vi "Web Server Startup.vi"(6 "LabVIEW Web Service":refnum<class "Web Service.lvclass">) -> ()   [LabVIEW 2026]
uses:
  <vilib>/wsapi/Web Service.lvclass
panel:
  # "Use the web service input terminal to call the VIs on the Service subpalette of the Web Services palette. Do not remove it from the connector pane unless you don't need access to the palette."
  # "Any additional terminals added to the connector pane of a startup VI will be ignored."
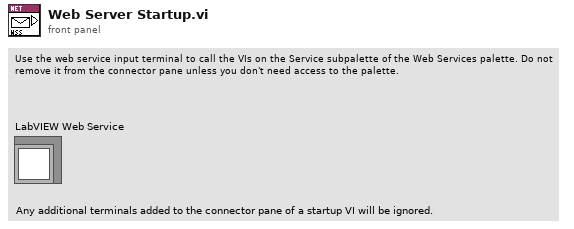
[diagram p1: front panel]
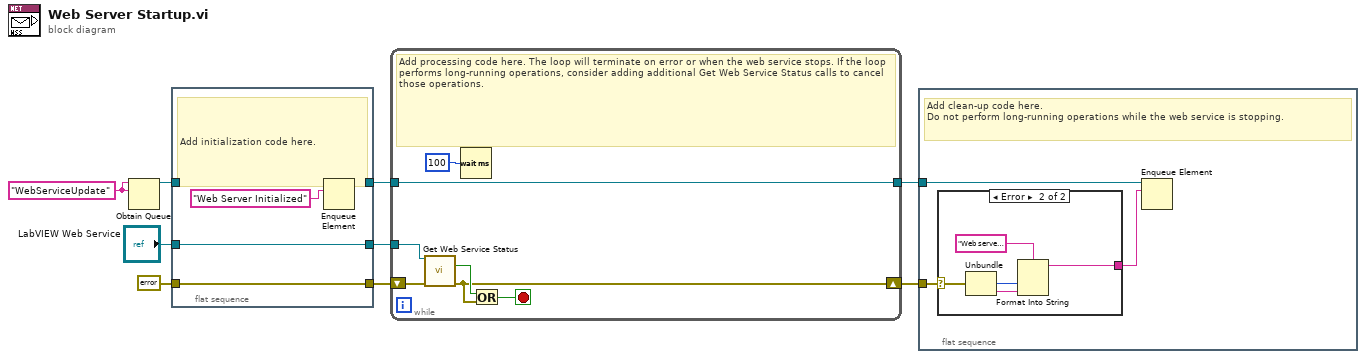
[diagram p0: block diagram]
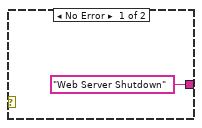
[diagram p2: hidden frame]
diagram:
  w4 = "WebServiceUpdate" ("name (unnamed)")
  n1 = Obtain Queue(name (unnamed)=w4, element data type=w4) -> (queue out=w3:refnum<queue>)  [unwired: 3 in, 2 out]
  n2 = flat-sequence {
    tunnel: "LabVIEW Web Service" -> [w14]
    tunnel: [w14] -> w8
    tunnel: [w12] -> w7
    tunnel: errorcluster {"status"=FALSE, "code"=0, "source"=""} ("error constant") -> [w12]
    tunnel: w3 -> [w13]
    tunnel: [w10] -> w1
    frame #0 {
      # "Add initialization code here."
      n3 = Enqueue Element(queue=w13, element="Web Server Initialized" ("name (unnamed)")) -> (queue out=w10:refnum<queue>)  [unwired: 2 in, 2 out]
    }
  }
  n4 = while {
    tunnel: w8 -> [w20]
    shift-right: [w17] -> w5
    shift-left: w7 -> [w18]
    tunnel: [w15] -> w2
    tunnel: w1 -> [w15]
    stop <- w19 stop-if-true
    # "Add processing code here. The loop will terminate on error or when the web service stops. If the loop performs long-running operations, consider adding additional Get Web Service Status calls to cancel those operations."
    n5 = call <vilib>:"Get Web Service Status.vi"("LabVIEW Web Service"=w20, "error in (no error)"=w18) -> ("service stopping?"=w21:bool, "error out"=w17:errorcluster)  [unwired: 11 in, 1 out]
    n6 = Wait (ms)(milliseconds to wait=u32 100) -> ()  [unwired: 1 out]
    n7 = Or(x=w21, y=w17) -> (x .or. y?=w19:bool)
  }
  n8 = flat-sequence {
    tunnel: w5 -> [w23]
    tunnel: w2 -> [w24]
    frame #0 {
      # "Add clean-up code here.\nDo not perform long-running operations while the web service is stopping."
      n9 = case shown="Error" w23 {
        selector: w23 -> [_ w29]
        tunnel: ["Web Server Shutdown" w26] -> w22
        frame No Error {
        }
        frame Error {
          n10 = Unbundle(w29) -> ("code"=w28:i32, "source"=w27:string)  [unwired: 1 out]
          n11 = Format Into String(format string="Web server terminated on error %d. Description: %s", w28, w27) -> (resulting string=w26:string)  [unwired: 2 in, 1 out]
        }
      }
      n12 = Enqueue Element(queue=w24, element=w22) -> ()  [unwired: 2 in, 3 out]
    }
  }
